vi "Voltage & Waveform.vi"() -> (0 "Bottom Rack Serial Number":string, 1 "Work Order":string, 2 "Waveform":u16(ring) items=["Sine", "Square"], 3 "Voltage":u16(ring) items=["3.3", "5.0", "12.0"], 4 "Frequency (MHz)":string, 6 "User":string, 8 "Work Order (Subnumber)":string, 9 "Top Rack Serial Number":string, 10 "PartNumber":string)   [LabVIEW 2024]
uses:
  <vilib>/regexp/Match Regular Expression.xnode
panel:
  in  "PartNumber":string
  in  "Top Rack Serial Number":string
  in  "User":string
  in  "Work Order":string
  in  "Frequency (MHz)":string
  in  "Bottom Rack Serial Number":string
  in  "Confirm":bool
  in  "Waveform":u16(ring) items=["Sine", "Square"]
  in  "Voltage":u16(ring) items=["3.3", "5.0", "12.0"]
  # "Please Select the Voltage and Waveform\nand Enter all Other Values"
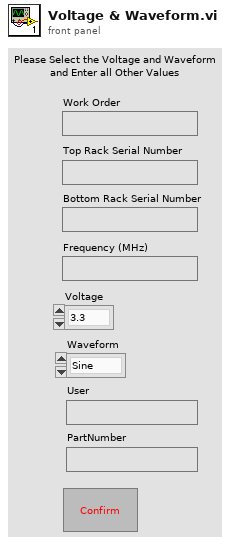
[diagram p1: front panel]
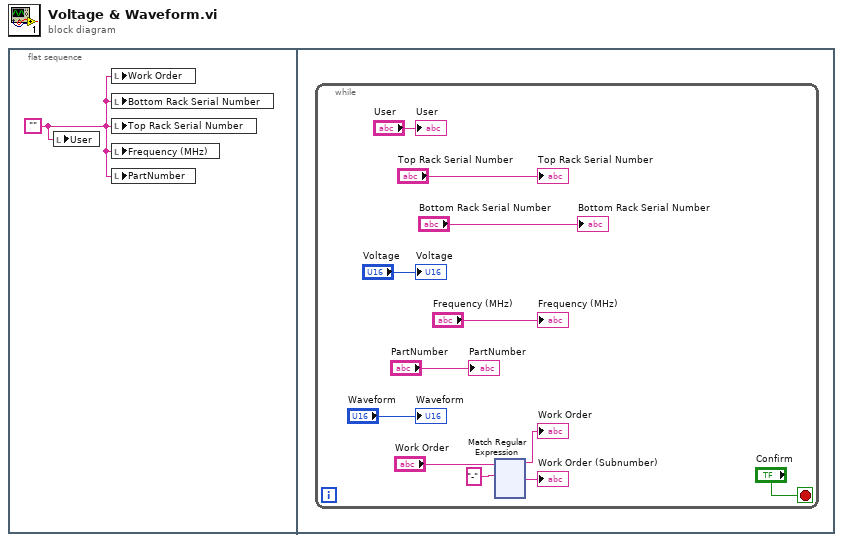
[diagram p0: block diagram]
diagram:
  n1 = flat-sequence {
    frame #0 {
      w1 = ""
      n2 = local write "User"(w1) -> ()
      n3 = local write "Work Order"(w1) -> ()
      n4 = local write "Bottom Rack Serial Number"(w1) -> ()
      n5 = local write "Top Rack Serial Number"(w1) -> ()
      n6 = local write "Frequency (MHz)"(w1) -> ()
      n7 = local write "PartNumber"(w1) -> ()
    }
    frame #1 {
      n8 = while {
        stop <- "Confirm" stop-if-true
        n9 = xnode "Match Regular Expression"("input string"="Work Order", "regular expression"="-") -> ("before match"=→"Work Order":string, "after match"=→"Work Order (Subnumber)":string)  [unwired: 4 in, 3 out]
        "Voltage" <- "Voltage"
        "Waveform" <- "Waveform"
        "User" <- "User"
        "Frequency (MHz)" <- "Frequency (MHz)"
        "Bottom Rack Serial Number" <- "Bottom Rack Serial Number"
        "Top Rack Serial Number" <- "Top Rack Serial Number"
        "PartNumber" <- "PartNumber"
      }
    }
  }
